vi "Main.vi"() -> ()   [LabVIEW 2023]
doc: "This template is for the Queued Message Handler design pattern.\n\nThe Event Handling Loop generates messages based on user interface actions.\n\nThe Message Handling Loop processes messages generated by the Event Handling Loop, or by other messages. The messages are string values, so new messages can be added easily to the Message Cases case structure in the Message Handling Loop. Each message cluster can also provide an optional value for Message Data, which is a variant that can be converted to whatever message-specific data is required."
uses:
  controls/UI Data.ctl
  support/Message Queue/Enqueue Message (Single).vi
  <vilib>/Utility/file.llb/Write Delimited Spreadsheet (string).vi
  <vilib>/Utility/file.llb/Write Delimited Spreadsheet (DBL).vi
  <vilib>/Instr/_visa.llb/VISA Configure Serial Port (Instr).vi
  <vilib>/Utility/error.llb/Error Cluster From Error Code.vi
  <vilib>/ErrorRing/Error Ring.xnode
  support/Message Queue/Message Queue.lvlib
  support/User Event - Stop/User Event - Stop.lvlib
panel:
  in  "File Path":path
  in  "Test Name":string
  out "Torque vs Displacement":cluster{dbl[], dbl[]}(graph)
  in  "VISA resource name":refnum<visa-resource-name>
  in  "Cycles":dbl
  in  "Torque":dbl
  in  "Microsteps":dbl
  in  "RPM":dbl
  in  "Clear":bool
  in  "Save":bool
  out "Status":string
  in  "Stop":bool
  in  "Start":bool
  in  "Exit":bool
  # "Torque vs Displacement"
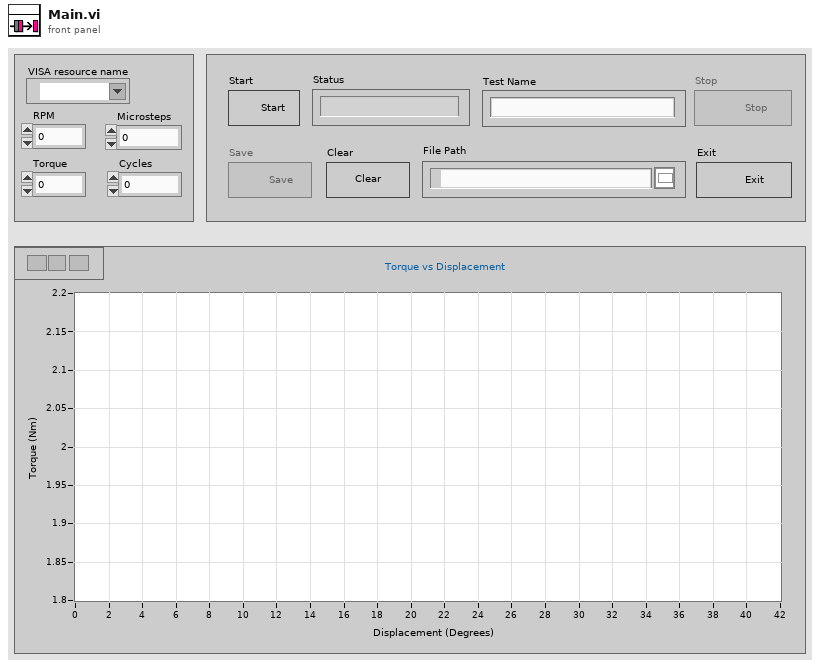
[diagram p1: front panel]
types:
  T1 = cluster{"RPM":dbl, "Microsteps":dbl, "Torque":dbl, "Cycles":dbl, "VISA resource name":refnum<visa-resource-name>}
  T2 = typedef "UI Data.ctl" = cluster{"Start ref":refnum<vi>, "Stop ref":refnum<vi>, "Status ref":refnum<vi>, "Exit ref":refnum<vi>, "Save ref":refnum<vi>, "Clear ref":refnum<vi>}
  T3 = typedef "Message Queue.lvlib/All Message Queues.ctl" = cluster{"UI":refnum<queue>, "Acquisition":refnum<queue>}
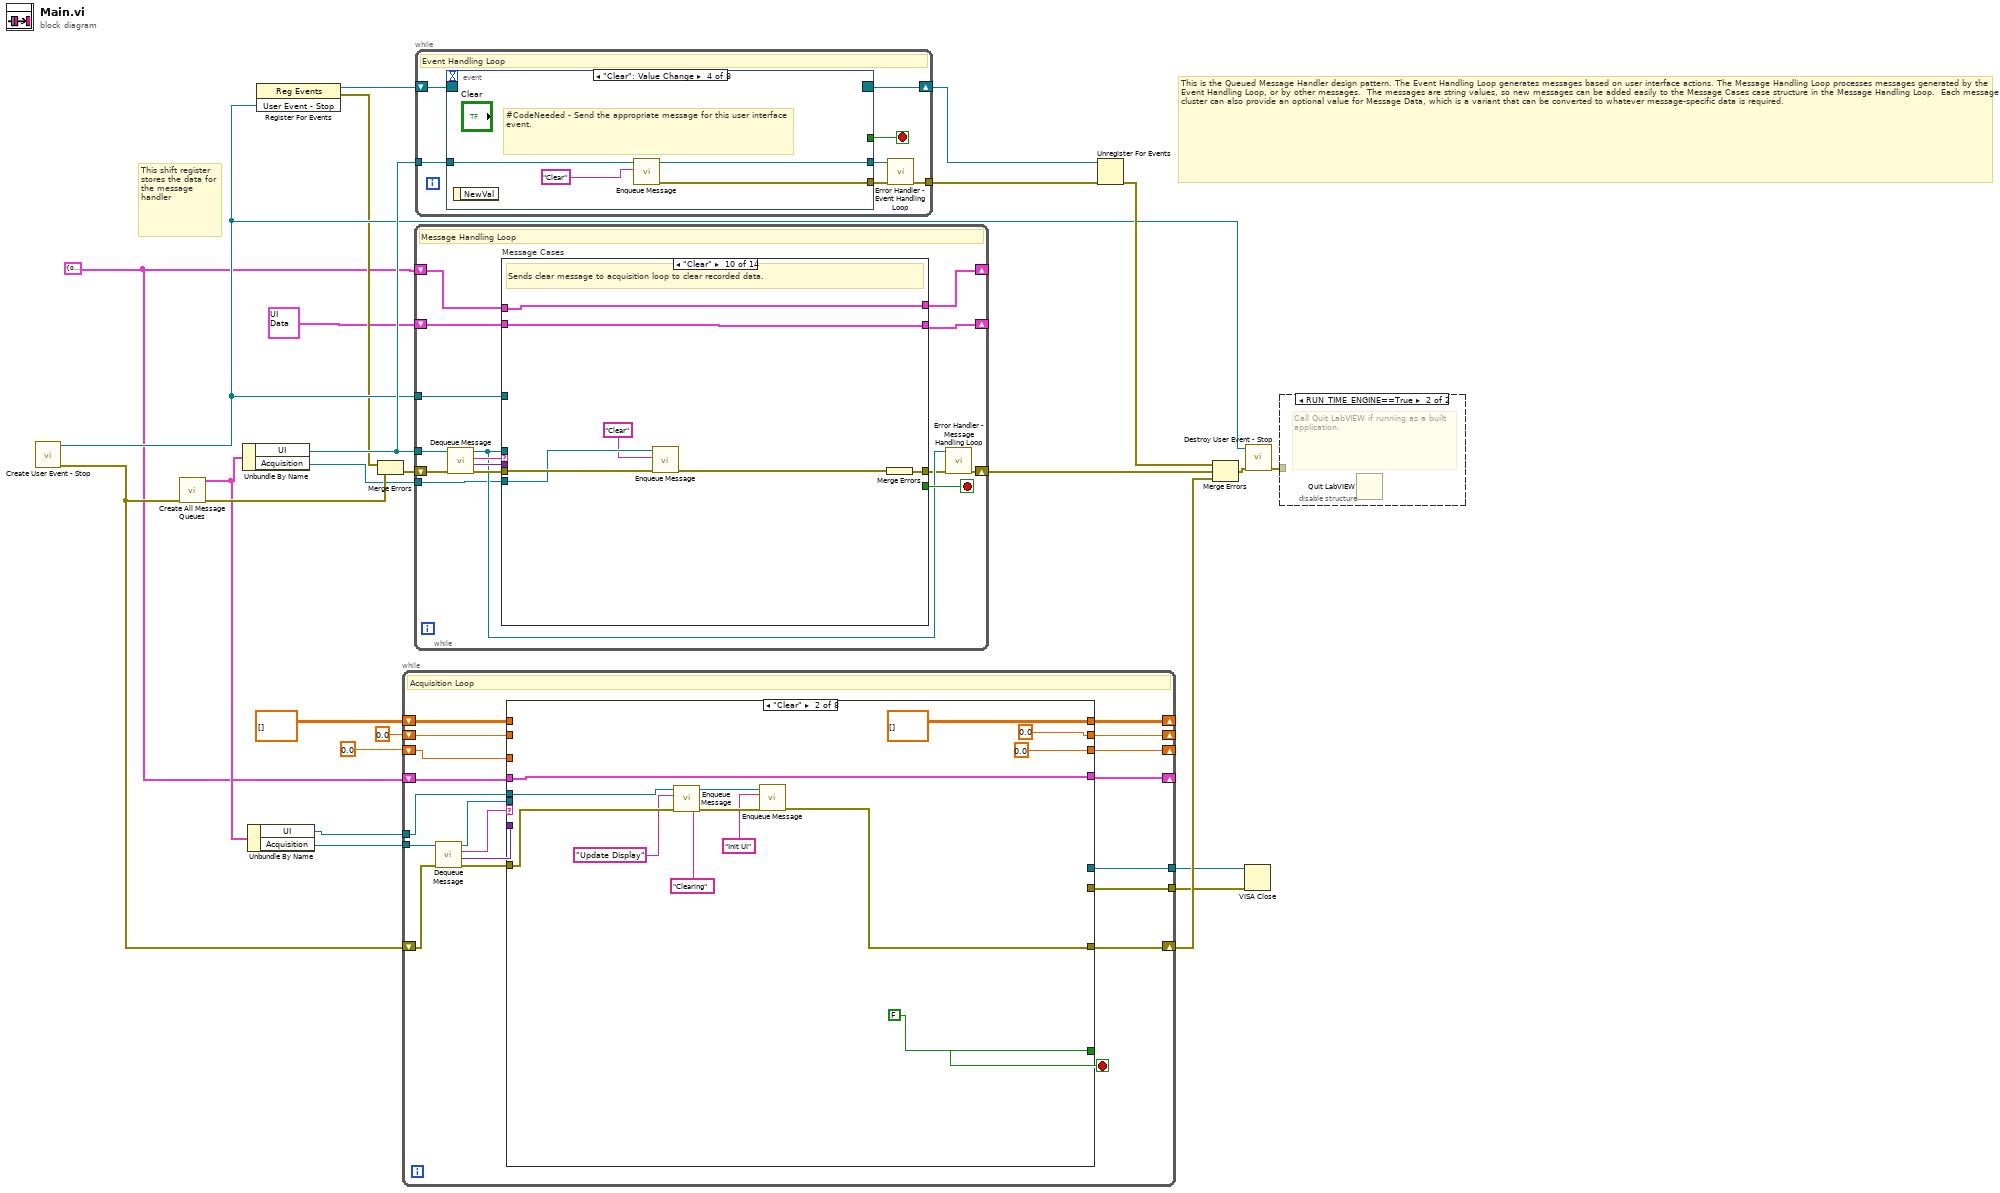
[diagram p0: block diagram]
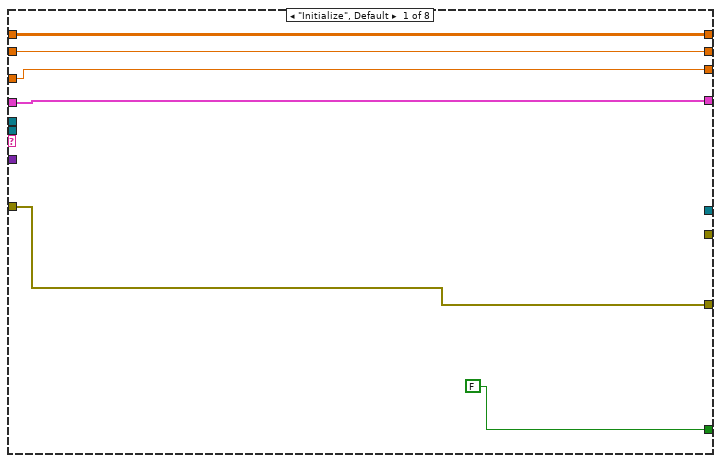
[diagram p2: hidden frame]
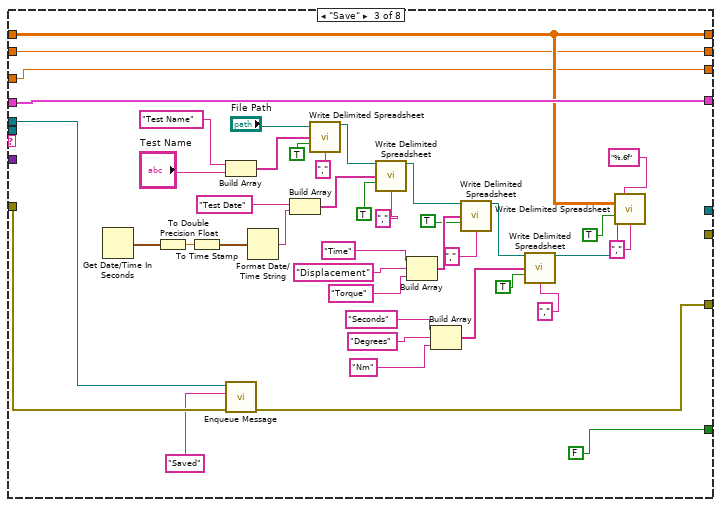
[diagram p3: hidden frame]
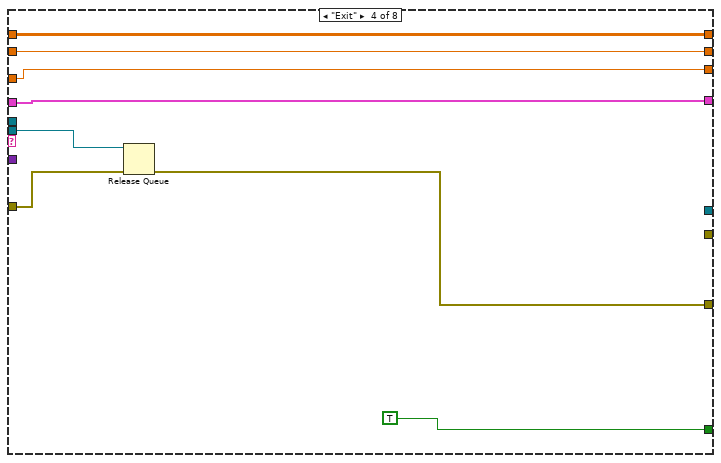
[diagram p4: hidden frame]
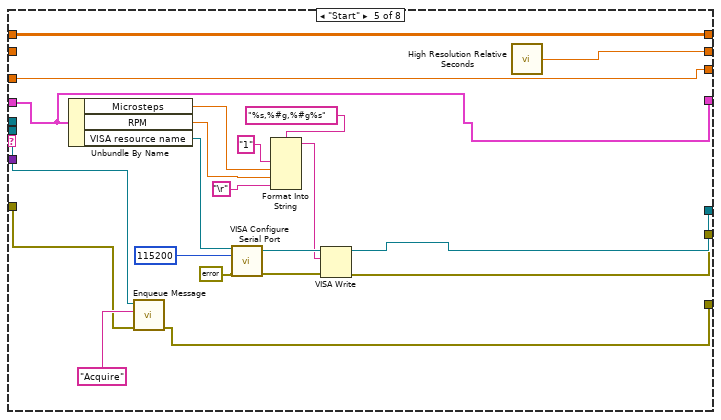
[diagram p5: hidden frame]
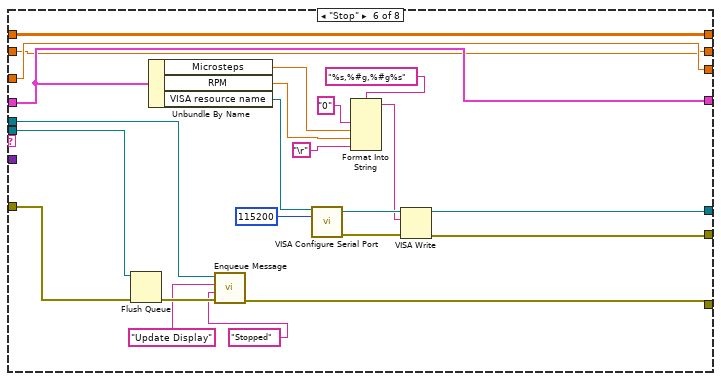
[diagram p6: hidden frame]
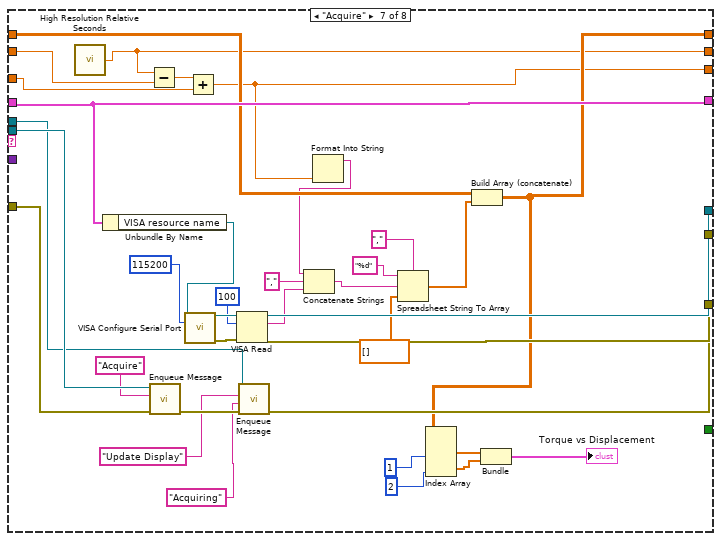
[diagram p7: hidden frame]
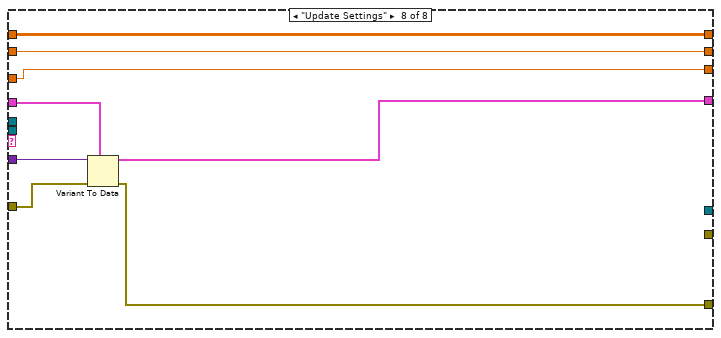
[diagram p8: hidden frame]
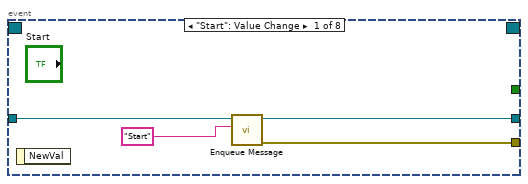
[diagram p10: hidden frame]
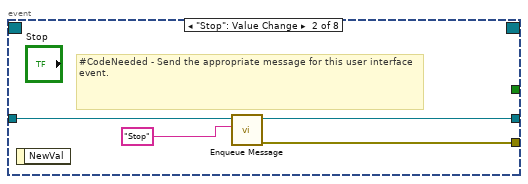
[diagram p11: hidden frame]
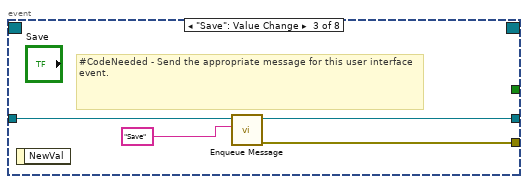
[diagram p12: hidden frame]
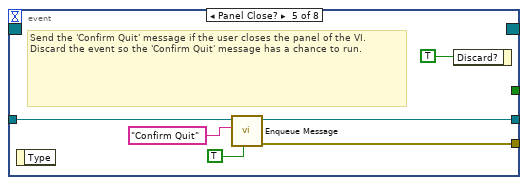
[diagram p13: hidden frame]
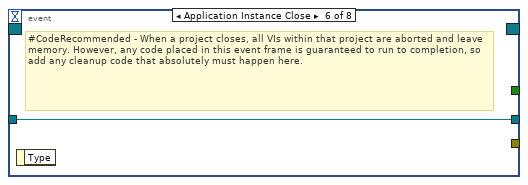
[diagram p14: hidden frame]
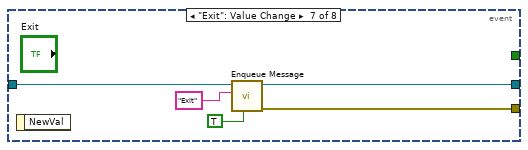
[diagram p15: hidden frame]
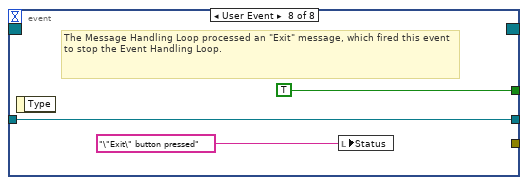
[diagram p16: hidden frame]
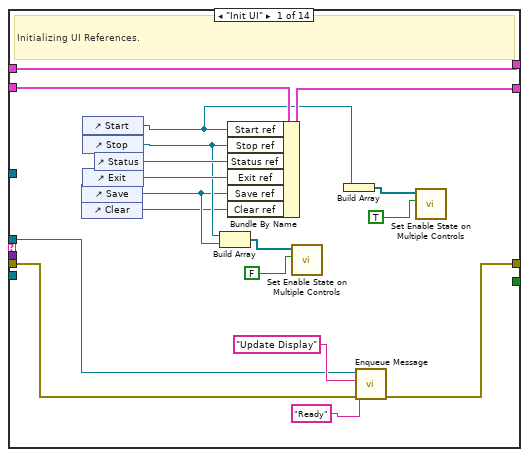
[diagram p17: hidden frame]
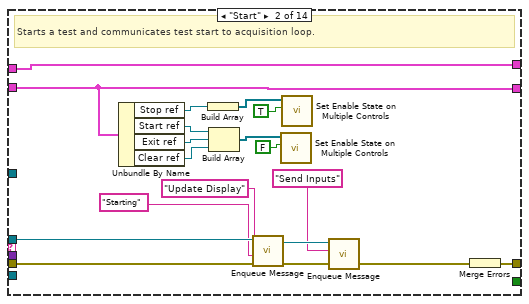
[diagram p18: hidden frame]
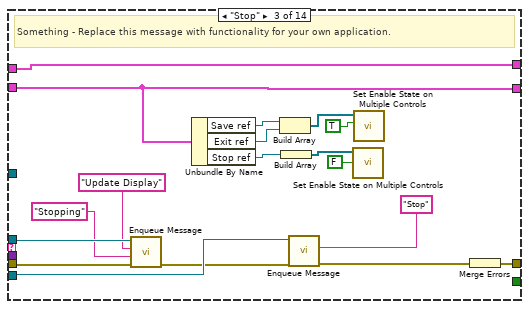
[diagram p19: hidden frame]
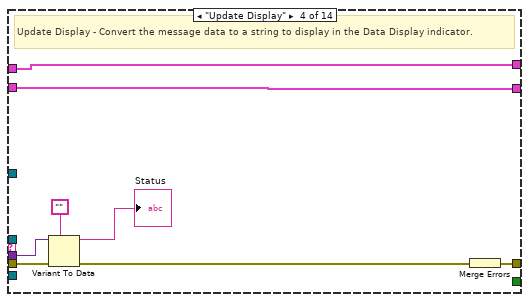
[diagram p20: hidden frame]
diagram:
  w8 = T1 {"RPM"=0.0, "Microsteps"=0.0, "Torque"=0.0, "Cycles"=0.0, "VISA resource name"=""}
  # "This is the Queued Message Handler design pattern. The Event Handling Loop generates messages based on user interface actions. The Message Handling Loop processes messages generated by the Event Handling Loop, or by other messages.  The messages are string values, so new messages can be added easily to the Message Cases case structure in the Message Handling Loop.  Each message cluster can also provide an optional value for Message Data, which is a variant that can be converted to whatever message-specific data is required."
  # "This shift register stores the data for the message handler"
  n1 = call "Create User Event - Stop.vi"() -> ("error out"=w9:errorcluster, "User Event - Stop"=w16:refnum<user-event>)  [unwired: 10 in]
  n2 = call "Create All Message Queues.vi"("error in (no error)"=w9) -> ("error out"=w25:errorcluster, "Message Queues out"=w11:T3)  [unwired: 9 in]
  n3 = Unbundle By Name(w11) -> ("UI"=w23:refnum<queue>, "Acquisition"=w12:refnum<queue>)
  n4 = Unbundle By Name(w11) -> ("UI"=w7:refnum<queue>, "Acquisition"=w10:refnum<queue>)
  n5 = register-events(w16) -> (reference out=w17:refnum<event-registration>, error out=w14:errorcluster)  [unwired: 2 in]
  n6 = Merge Errors(w14, w25) -> (w15:errorcluster)
  n7 = while {
    tunnel: w10 -> [w44]
    shift-right: [w32] -> w6
    shift-left: w9 -> [w43]
    shift-right: [w38] -> _
    shift-left: w8 -> [w41]
    tunnel: w7 -> [w33]
    tunnel: [w35] -> w5
    tunnel: [w34] -> w4
    shift-right: [w30] -> _
    shift-left: dbl[][] [] -> [w31]
    shift-right: [w29] -> _
    shift-left: 0.0 -> [w28]
    shift-right: [w27] -> _
    shift-left: 0.0 -> [w26]
    stop <- w37 stop-if-true
    # "Acquisition Loop"
    n8 = call "Dequeue Message.vi"("error in (no error)"=w43, "Message Queue"=w44) -> ("error out"=w42:errorcluster, "Message Data"=w39:variant, "Message"=w40:string, "dup Message Queue"=w36:refnum<queue>)  [unwired: 6 in]
    n9 = case shown="\"Clear\"" w40 {
      tunnel: w42 -> [w48 w61 w102 w110 w121 w142 w185 w199]
      tunnel: w41 -> [w50 w63 w105 w113 w124 w147 w191 w200]
      tunnel: w39 -> [_ _ _ _ _ _ _ w201]
      tunnel: [w50 w63 w105 w113 w124 w147 w191 w198] -> w38
      tunnel: [FALSE FALSE FALSE TRUE _ _ _ _] -> w37
      tunnel: w36 -> [_ _ _ w111 w118 w143 w186 _]
      tunnel: [_ _ _ _ w122 w146 w188 _] -> w35
      tunnel: [_ _ _ _ w120 w145 w187 _] -> w34
      tunnel: w33 -> [_ w60 w103 _ _ w139 w181 _]
      tunnel: [w48 w55 w64 w109 w117 w140 w182 w197] -> w32
      tunnel: w31 -> [w47 _ w97 w108 w116 w144 w174 w196]
      tunnel: [w47 dbl[][] [] w97 w108 w116 w144 w163 w196] -> w30
      tunnel: [w46 0.0 w78 w107 w115 w137 w159 w195] -> w29
      tunnel: w28 -> [w46 _ w78 w107 w115 w137 w162 w195]
      tunnel: [w45 0.0 w75 w106 w114 w136 w158 w194] -> w27
      tunnel: w26 -> [w45 _ w75 w106 _ w136 w161 w194]
      frame "Initialize", Default {
      }
      frame "Clear" {
        n10 = call-poly "Enqueue Message.vi"("error in (no error)"=w61, "Message Data"="Clearing" ("Message"), "Message"="Update Display", "Message Queue"=w60) -> ("error out"=w56:errorcluster, "dup Message Queue"=w57:refnum<queue>)  [unwired: 6 in]
        n11 = call-poly "Enqueue Message.vi"("error in (no error)"=w56, "Message"="Init UI", "Message Queue"=w57) -> ("error out"=w55:errorcluster)  [unwired: 7 in, 1 out]
      }
      frame "Save" {
        n12 = Get Date/Time In Seconds() -> (seconds since 1Jan1904=w73:timestamp)
        n13 = To Double Precision Float(number=w73) -> (double precision float=w74:dbl)
        n14 = To Time Stamp(1:w74) -> (0:w70:timestamp)
        n15 = Build Array("Test Name" ("delimiter (\\t)"), "Test Name") -> (w95:string[])
        n16 = call-poly "Enqueue Message.vi"("error in (no error)"=w102, "Message"="Saved", "Message Queue"=w103) -> ("error out"=w64:errorcluster)  [unwired: 7 in, 1 out]
        n17 = Format Date/Time String(seconds (now)=w70) -> (date/time string=w66:string)  [unwired: 2 in]
        n18 = Build Array("Test Date" ("delimiter (\\t)"), w66) -> (w65:string[])
        n19 = call-poly <vilib>:"Write Delimited Spreadsheet.vi"("file path (dialog if empty)"="File Path", "1D data"=w95, "append to file? (new file:F)"=TRUE, "delimiter (\\t)"="," ("delimiter (\\t)")) -> ("new file path (Not A Path if cancelled)"=w69:path)  [unwired: 10 in, 1 out]
        n20 = call-poly <vilib>:"Write Delimited Spreadsheet.vi"("file path (dialog if empty)"=w69, "1D data"=w65, "append to file? (new file:F)"=TRUE, "delimiter (\\t)"="," ("delimiter (\\t)")) -> ("new file path (Not A Path if cancelled)"=w68:path)  [unwired: 10 in, 1 out]
        n21 = Build Array("Time" ("element"), "Displacement" ("delimiter (\\t)"), "Torque" ("delimiter (\\t)")) -> (w89:string[])
        n22 = Build Array("Seconds" ("element"), "Degrees" ("delimiter (\\t)"), "Nm" ("delimiter (\\t)")) -> (w88:string[])
        n23 = call-poly <vilib>:"Write Delimited Spreadsheet.vi"("file path (dialog if empty)"=w68, "1D data"=w89, "append to file? (new file:F)"=TRUE, "delimiter (\\t)"="," ("delimiter (\\t)")) -> ("new file path (Not A Path if cancelled)"=w87:path)  [unwired: 10 in, 1 out]
        n24 = call-poly <vilib>:"Write Delimited Spreadsheet.vi"("file path (dialog if empty)"=w87, "1D data"=w88, "append to file? (new file:F)"=TRUE, "delimiter (\\t)"="," ("delimiter (\\t)")) -> ("new file path (Not A Path if cancelled)"=w86:path)  [unwired: 10 in, 1 out]
        n25 = call-poly <vilib>:"Write Delimited Spreadsheet.vi"("file path (dialog if empty)"=w86, "format (%.3f)"="%.6f", "2D data"=w97, "append to file? (new file:F)"=TRUE, "delimiter (\\t)"="," ("delimiter (\\t)")) -> ()  [unwired: 9 in, 2 out]
      }
      frame "Exit" {
        n26 = Release Queue(queue=w111, error in (no error)=w110) -> (error out=w109:errorcluster)  [unwired: 1 in, 2 out]
      }
      frame "Start" {
        n27 = Unbundle By Name(w124) -> ("Microsteps"=w131:dbl, "RPM"=w130:dbl, "VISA resource name"=w129:refnum<visa-resource-name>)
        n28 = call-poly "Enqueue Message.vi"("error in (no error)"=w121, "Message"="Acquire", "Message Queue"=w118) -> ("error out"=w117:errorcluster)  [unwired: 7 in, 1 out]
        n29 = call-poly "VISA Configure Serial Port"("VISA resource name"=w129, "baud rate (9600)"=u32 115200, "error in (no error)"=errorcluster {"status"=FALSE, "code"=0, "source"=""}) -> ("VISA resource name out"=w126:refnum<visa-resource-name>, "error out"=w127:errorcluster)  [unwired: 11 in]
        n30 = Format Into String(format string="%s,%#g,%#g%s", "1", w131, w130, "\r") -> (resulting string=w125:string)  [unwired: 2 in, 1 out]
        n31 = VISA Write(VISA resource name=w126, write buffer=w125, error in (no error)=w127) -> (VISA resource name out=w122:refnum<visa-resource-name>, error out=w120:errorcluster)  [unwired: 1 out]
        n32 = call <vilib>:"High Resolution Relative Seconds.vi"() -> ("relative seconds"=w114:dbl)
      }
      frame "Stop" {
        n33 = Flush Queue(queue=w143, error in (no error)=w142) -> (error out=w141:errorcluster)  [unwired: 2 out]
        n34 = Unbundle By Name(w147) -> ("Microsteps"=w154:dbl, "RPM"=w153:dbl, "VISA resource name"=w152:refnum<visa-resource-name>)
        n35 = call-poly "Enqueue Message.vi"("error in (no error)"=w141, "Message Data"="Stopped" ("Message"), "Message"="Update Display", "Message Queue"=w139) -> ("error out"=w140:errorcluster)  [unwired: 6 in, 1 out]
        n36 = call-poly "VISA Configure Serial Port"("VISA resource name"=w152, "baud rate (9600)"=u32 115200) -> ("VISA resource name out"=w149:refnum<visa-resource-name>, "error out"=w150:errorcluster)  [unwired: 12 in]
        n37 = Format Into String(format string="%s,%#g,%#g%s", "0", w154, w153, "\r") -> (resulting string=w148:string)  [unwired: 2 in, 1 out]
        n38 = VISA Write(VISA resource name=w149, write buffer=w148, error in (no error)=w150) -> (VISA resource name out=w146:refnum<visa-resource-name>, error out=w145:errorcluster)  [unwired: 1 out]
      }
      frame "Acquire" {
        n39 = call <vilib>:"High Resolution Relative Seconds.vi"() -> ("relative seconds"=w158:dbl)
        n40 = Unbundle By Name(w191) -> ("VISA resource name"=w193:refnum<visa-resource-name>)
        n41 = Subtract(x=w158, y=w161) -> (x-y=w160:dbl)
        n42 = call-poly "Enqueue Message.vi"("error in (no error)"=w185, "Message"="Acquire", "Message Queue"=w186) -> ("error out"=w183:errorcluster)  [unwired: 7 in, 1 out]
        n43 = call-poly "VISA Configure Serial Port"("VISA resource name"=w193, "baud rate (9600)"=u32 115200) -> ("VISA resource name out"=w190:refnum<visa-resource-name>, "error out"=w189:errorcluster)  [unwired: 12 in]
        n44 = Add(x=w160, y=w162) -> (x+y=w159:dbl)
        n45 = VISA Read(VISA resource name=w190, byte count=u32 100, error in (no error)=w189) -> (VISA resource name out=w188:refnum<visa-resource-name>, read buffer=w165:string, error out=w187:errorcluster)  [unwired: 1 out]
        n46 = call-poly "Enqueue Message.vi"("error in (no error)"=w183, "Message Data"="Acquiring" ("\"Do Something\" button pressed"), "Message"="Update Display", "Message Queue"=w181) -> ("error out"=w182:errorcluster)  [unwired: 6 in, 1 out]
        n47 = Format Into String(w159) -> (resulting string=w164:string)  [unwired: 3 in, 1 out]
        n48 = Concatenate Strings(w164, "," ("string"), w165) -> (w166:string)
        n49 = Spreadsheet String To Array(delimiter (Tab)=",", format string="%d", spreadsheet string=w166, array type (2D Dbl)=dbl[] []) -> (array=w173:dbl[])
        n50 = Build Array (concatenate)(w174, w173) -> (w163:dbl[][])
        n51 = Index Array(array=w163, index (col) #1=1 ("index (col)"), index (col) #2=2 ("index (col)")) -> (element #1=w170:dbl[], element #2=w169:dbl[])  [unwired: 2 in]
        n52 = Bundle(w170, w169) -> (→"Torque vs Displacement":cluster{dbl[], dbl[]})  [unwired: 1 in]
      }
      frame "Update Settings" {
        n53 = Variant To Data(error in=w199, type=w200, Variant=w201) -> (data=w198:T1, error out=w197:errorcluster)
      }
    }
  }
  n54 = while {
    tunnel: w23 -> [w208]
    shift-right: [w215] -> _
    shift-left: T2 {"Start ref"=refnum, "Stop ref"=refnum, "Status ref"=refnum, "Exit ref"=refnum, "Save ref"=refnum, "Clear ref"=refnum} ("Data Cluster") -> [w216]
    tunnel: w16 -> [w213]
    shift-right: [w204] -> _
    shift-left: w8 -> [w203]
    tunnel: w12 -> [w202]
    shift-right: [w206] -> w24
    shift-left: w15 -> [w212]
    stop <- w214 stop-if-true
    # "Message Handling Loop"
    n55 = call "Dequeue Message.vi"("error in (no error)"=w212, "Message Queue"=w208) -> ("error out"=w211:errorcluster, "Message Data"=w209:variant, "Message"=w210:string, "dup Message Queue"=w207:refnum<queue>)  [unwired: 6 in]
    n56 = case "Message Cases" shown="\"Clear\"" w210 {
      selector: w210 -> [_ _ _ _ _ _ _ _ _ _ _ _ _ w364]
      tunnel: w207 -> [w226 w251 w264 _ _ w291 _ w303 w315 _ _ _ w362 _]
      tunnel: w211 -> [w225 w252 w266 w277 w287 w295 w299 w304 w316 w323 w330 w342 w355 _]
      tunnel: [w234 w253 w271 w278 w281 w293 w297 w313 w319 w326 w333 w349 w358 w365] -> w205
      tunnel: w216 -> [w233 w241 w255 w279 w286 w294 w298 w305 w320 w327 w334 w350 w361 w366]
      tunnel: [w232 w241 w255 w279 w286 w294 w298 w305 w320 w327 w334 w350 w361 w366] -> w215
      tunnel: [_ _ _ _ _ _ _ _ _ _ _ _ TRUE _] -> w214
      tunnel: w209 -> [_ _ _ w276 w285 _ _ _ _ _ _ _ _ _]
      tunnel: w213 -> [_ _ _ _ _ _ _ _ _ _ _ _ w357 _]
      tunnel: w203 -> [w227 w248 w270 w272 w280 w288 w296 w312 w318 w325 w332 w348 w351 w363]
      tunnel: [w227 w248 w270 w272 w280 w288 w296 w312 w318 w325 w332 w341 w351 w363] -> w204
      tunnel: w202 -> [_ _ w267 _ _ _ _ _ _ w322 w329 w339 w354 _]
      frame "Init UI" {
        # "Initializing UI References."
        n57 = control-ref of="Save"() -> (w221:refnum<vi>)
        n58 = control-ref of="Clear"() -> (w220:refnum<vi>)
        n59 = control-ref of="Start"() -> (w217:refnum<vi>)
        n60 = control-ref of="Stop"() -> (w222:refnum<vi>)
        n61 = control-ref of="Exit"() -> (w230:refnum<vi>)
        n62 = control-ref of="Status"() -> (w231:refnum<vi>)
        n63 = Build Array(w222, w221) -> (w223:refnum<vi>[])
        n64 = Bundle By Name(cluster=w233, "Start ref"=w217, "Stop ref"=w222, "Status ref"=w231, "Exit ref"=w230, "Save ref"=w221, "Clear ref"=w220) -> (w232:T2)
        n65 = call "Set Enable State on Multiple Controls.vi"("Enable?"=FALSE, "Controls"=w223) -> ()  [unwired: 10 in]
        n66 = Build Array(w217) -> (w218:refnum<vi>[])
        n67 = call-poly "Enqueue Message.vi"("error in (no error)"=w225, "Message Data"="Ready" ("Initial Message"), "Message"="Update Display", "Message Queue"=w226) -> ("error out"=w234:errorcluster)  [unwired: 6 in, 1 out]
        n68 = call "Set Enable State on Multiple Controls.vi"("Enable?"=TRUE, "Controls"=w218) -> ()  [unwired: 10 in]
      }
      frame "Start" {
        # "Starts a test and communicates test start to acquisition loop."
        n69 = Unbundle By Name(w241) -> ("Stop ref"=w238:refnum<vi>, "Start ref"=w236:refnum<vi>, "Exit ref"=w240:refnum<vi>, "Clear ref"=w235:refnum<vi>)
        n70 = Build Array(w238) -> (w237:refnum<vi>[])
        n71 = Build Array(w236, w240, w235) -> (w242:refnum<vi>[])
        n72 = call-poly "Enqueue Message.vi"("error in (no error)"=w252, "Message Data"="Starting" ("\"Do Something\" button pressed"), "Message"="Update Display", "Message Queue"=w251) -> ("error out"=w247:errorcluster, "dup Message Queue"=w246:refnum<queue>)  [unwired: 6 in]
        n73 = call "Set Enable State on Multiple Controls.vi"("Enable?"=FALSE, "Controls"=w242) -> ()  [unwired: 10 in]
        n74 = call "Set Enable State on Multiple Controls.vi"("Enable?"=TRUE, "Controls"=w237) -> ()  [unwired: 10 in]
        n75 = call-poly "Enqueue Message.vi"("error in (no error)"=w247, "Message"="Send Inputs", "Message Queue"=w246) -> ("error out"=w244:errorcluster)  [unwired: 7 in, 1 out]
        n76 = Merge Errors(w244) -> (w253:errorcluster)
      }
      frame "Stop" {
        # "Something - Replace this message with functionality for your own application."
        n77 = call-poly "Enqueue Message.vi"("error in (no error)"=w266, "Message Data"="Stopping" ("Message"), "Message"="Update Display", "Message Queue"=w264) -> ("error out"=w265:errorcluster)  [unwired: 6 in, 1 out]
        n78 = Unbundle By Name(w255) -> ("Save ref"=w260:refnum<vi>, "Exit ref"=w254:refnum<vi>, "Stop ref"=w259:refnum<vi>)
        n79 = Build Array(w260, w254) -> (w261:refnum<vi>[])
        n80 = Build Array(w259) -> (w258:refnum<vi>[])
        n81 = call-poly "Enqueue Message.vi"("error in (no error)"=w265, "Message"="Stop", "Message Queue"=w267) -> ("error out"=w269:errorcluster)  [unwired: 7 in, 1 out]
        n82 = call "Set Enable State on Multiple Controls.vi"("Enable?"=FALSE, "Controls"=w258) -> ()  [unwired: 10 in]
        n83 = call "Set Enable State on Multiple Controls.vi"("Enable?"=TRUE, "Controls"=w261) -> ()  [unwired: 10 in]
        n84 = Merge Errors(w269) -> (w271:errorcluster)
      }
      frame "Update Display" {
        # "Update Display - Convert the message data to a string to display in the Data Display indicator."
        n85 = Variant To Data(error in=w277, type="", Variant=w276) -> (data=→"Status":string, error out=w274:errorcluster)
        n86 = Merge Errors(w274) -> (w278:errorcluster)
      }
      frame "Error" {
        # "Error - Display an error dialog. This message is sent by the \"Error Handler\" VIs at the end of other loops in this application."
        n87 = Variant To Data(error in=w287, type=errorcluster {"status"=FALSE, "code"=0, "source"=""} ("error constant"), Variant=w285) -> (data=w283:errorcluster, error out=w282:errorcluster)
        n88 = call <vilib>:"Simple Error Handler.vi"("error in (no error)"=w283) -> ()  [unwired: 4 in, 5 out]
        n89 = Merge Errors(w282) -> (w281:errorcluster)
      }
      frame "Confirm Quit" {
        # "#CodeNeeded - If you want to provide an \"Are you sure\" dialog (or some other notification) before the application exits, place that code here. This message is typically sent from a Panel Close? event."
        # "Confirm Quit - Message that can confirm whether or not the user wants to exit the application."
        n90 = call-poly "Enqueue Message.vi"("Priority Message? (F)"=TRUE, "error in (no error)"=w295, "Message"="Exit", "Message Queue"=w291) -> ("error out"=w292:errorcluster)  [unwired: 6 in, 1 out]
        n91 = Merge Errors(w292) -> (w293:errorcluster)
      }
      frame "---Copy This Frame---" {
        # "Duplicate this frame when creating new messages.  Change this comment in the duplicated frame to describe this message."
        n92 = Merge Errors(w299) -> (w297:errorcluster)
      }
      frame "Saved" {
        # "Duplicate this frame when creating new messages.  Change this comment in the duplicated frame to describe this message."
        n93 = call-poly "Enqueue Message.vi"("error in (no error)"=w304, "Message Data"="Saved" ("Message"), "Message"="Update Display", "Message Queue"=w303) -> ("error out"=w300:errorcluster)  [unwired: 6 in, 1 out]
        n94 = Unbundle By Name(w305) -> ("Clear ref"=w311:refnum<vi>, "Save ref"=w309:refnum<vi>)
        n95 = Build Array(w311) -> (w308:refnum<vi>[])
        n96 = Build Array(w309) -> (w310:refnum<vi>[])
        n97 = call "Set Enable State on Multiple Controls.vi"("Enable?"=TRUE, "Controls"=w308) -> ()  [unwired: 10 in]
        n98 = call "Set Enable State on Multiple Controls.vi"("Enable?"=FALSE, "Controls"=w310) -> ()  [unwired: 10 in]
        n99 = Merge Errors(w300) -> (w313:errorcluster)
      }
      frame "Initialize" {
        # "Duplicate this frame when creating new messages.  Change this comment in the duplicated frame to describe this message."
        n100 = call-poly "Enqueue Message.vi"("error in (no error)"=w316, "Message"="Init UI", "Message Queue"=w315) -> ("error out"=w317:errorcluster)  [unwired: 7 in, 1 out]
        n101 = Merge Errors(w317) -> (w319:errorcluster)
      }
      frame "Clear" {
        # "Sends clear message to acquisition loop to clear recorded data."
        n102 = call-poly "Enqueue Message.vi"("error in (no error)"=w323, "Message"="Clear", "Message Queue"=w322) -> ("error out"=w324:errorcluster)  [unwired: 7 in, 1 out]
        n103 = Merge Errors(w324) -> (w326:errorcluster)
      }
      frame "Save" {
        # "Saves Current Data"
        n104 = call-poly "Enqueue Message.vi"("error in (no error)"=w330, "Message"="Save", "Message Queue"=w329) -> ("error out"=w331:errorcluster)  [unwired: 7 in, 1 out]
        n105 = Merge Errors(w331) -> (w333:errorcluster)
      }
      frame "Send Inputs" {
        # "Send updated inputs to acquistion loop."
        n106 = Bundle By Name(cluster=w348, "RPM"="RPM", "Microsteps"="Microsteps", "Torque"="Torque", "Cycles"="Cycles", "VISA resource name"="VISA resource name") -> (w341:T1)
        n107 = call-poly "Enqueue Message.vi"("error in (no error)"=w342, "Message Data"=w341, "Message"="Update Settings", "Message Queue"=w339) -> ("error out"=w337:errorcluster, "dup Message Queue"=w335:refnum<queue>)  [unwired: 6 in]
        n108 = call-poly "Enqueue Message.vi"("error in (no error)"=w337, "Message"="Start", "Message Queue"=w335) -> ("error out"=w336:errorcluster)  [unwired: 7 in, 1 out]
        n109 = Merge Errors(w336) -> (w349:errorcluster)
      }
      frame "Exit" {
        # "Stop the VI"
        # "Release the message queue reference"
        # "Exit - Exit the application."
        n110 = call-poly "Enqueue Message.vi"("Priority Message? (F)"=TRUE, "Message"="Exit", "Message Queue"=w354) -> ()  [unwired: 7 in, 2 out]
        n111 = call "Fire User Event - Stop.vi"("User Event - Stop"=w357) -> ("error out"=w356:errorcluster)  [unwired: 10 in]
        n112 = Release Queue(queue=w362, error in (no error)=w355) -> (error out=w359:errorcluster)  [unwired: 1 in, 2 out]
        n113 = Merge Errors(w356, w359) -> (w358:errorcluster)
      }
      frame Default {
        # "'Default' case only runs if there is a message that isn't defined in any of the other cases.  Output a programming error."
        n114 = xnode "Error Ring"("parameter 0"=w364) -> ("error out"=w365:errorcluster)
      }
    }
    n115 = call "Error Handler - Message Handling Loop.vi"("error in (no error)"=w205, "Message Queue"=w207) -> ("dup error in"=w206:errorcluster)  [unwired: 8 in, 1 out]
  }
  n116 = while {
    tunnel: w23 -> [w380]
    shift-right: [w378] -> w20
    shift-left: w17 -> [w379]
    tunnel: [w374] -> w18
    stop <- w376 stop-if-true
    # "Event Handling Loop"
    n117 = event shown="[3] \"Clear\": Value Change" {
      selector: w379 -> [_ _ _ _ _ _ _ _]
      dyn-events: [_ _ _ _ _ _ _ _] -> w378
      timeout: _ -> [_ _ _ _ _ _ _ _]
      tunnel: [_ _ _ _ _ _ _ TRUE ("Discard?")] -> w376
      tunnel: w380 -> [w384 w388 w392 w396 w401 w403 w408 w411]
      tunnel: [w381 w385 w389 w393 w400 _ w407 _] -> w377
      tunnel: [w383 w387 w391 w395 w399 w403 w406 w411] -> w375
      event "Start": Value Change {
        n118 = event-data() -> ()  [unwired: 1 in, 1 out]
        n119 = call-poly "Enqueue Message.vi"("Message"="Start", "Message Queue"=w384) -> ("error out"=w381:errorcluster, "dup Message Queue"=w383:refnum<queue>)  [unwired: 8 in]
      }
      event "Stop": Value Change {
        # "#CodeNeeded - Send the appropriate message for this user interface event."
        n120 = event-data() -> ()  [unwired: 1 in, 1 out]
        n121 = call-poly "Enqueue Message.vi"("Message"="Stop", "Message Queue"=w388) -> ("error out"=w385:errorcluster, "dup Message Queue"=w387:refnum<queue>)  [unwired: 8 in]
      }
      event "Save": Value Change {
        # "#CodeNeeded - Send the appropriate message for this user interface event."
        n122 = event-data() -> ()  [unwired: 1 in, 1 out]
        n123 = call-poly "Enqueue Message.vi"("Message"="Save", "Message Queue"=w392) -> ("error out"=w389:errorcluster, "dup Message Queue"=w391:refnum<queue>)  [unwired: 8 in]
      }
      event "Clear": Value Change {
        # "#CodeNeeded - Send the appropriate message for this user interface event."
        n124 = event-data() -> ()  [unwired: 1 in, 1 out]
        n125 = call-poly "Enqueue Message.vi"("Message"="Clear", "Message Queue"=w396) -> ("error out"=w393:errorcluster, "dup Message Queue"=w395:refnum<queue>)  [unwired: 8 in]
      }
      event Panel Close? {
        # "Send the 'Confirm Quit' message if the user closes the panel of the VI. Discard the event so the 'Confirm Quit' message has a chance to run."
        n126 = event-data() -> ()  [unwired: 1 in, 1 out]
        n127 = call-poly "Enqueue Message.vi"("Priority Message? (F)"=TRUE, "Message"="Confirm Quit", "Message Queue"=w401) -> ("error out"=w400:errorcluster, "dup Message Queue"=w399:refnum<queue>)  [unwired: 7 in]
        n128 = event-data("Discard?"=TRUE) -> ()  [unwired: 1 in, 1 out]
      }
      event Application Instance Close {
        # "#CodeRecommended - When a project closes, all VIs within that project are aborted and leave memory. However, any code placed in this event frame is guaranteed to run to completion, so add any cleanup code that absolutely must happen here."
        n129 = event-data() -> ()  [unwired: 1 in, 1 out]
      }
      event "Exit": Value Change {
        n130 = event-data() -> ()  [unwired: 1 in, 1 out]
        n131 = call-poly "Enqueue Message.vi"("Priority Message? (F)"=TRUE, "Message"="Exit", "Message Queue"=w408) -> ("error out"=w407:errorcluster, "dup Message Queue"=w406:refnum<queue>)  [unwired: 7 in]
      }
      event User Event {
        # "The Message Handling Loop processed an \"Exit\" message, which fired this event to stop the Event Handling Loop."
        n132 = event-data() -> ()  [unwired: 1 in, 1 out]
        n133 = local write "Status"("\"Exit\" button pressed" ("VI Stopped")) -> ()
      }
    }
    n134 = call "Error Handler - Event Handling Loop.vi"("error in (no error)"=w377, "Message Queue"=w375) -> ("dup error in"=w374:errorcluster)  [unwired: 8 in, 1 out]
  }
  n135 = Unregister For Events(event registration refnum=w20, error in=w18) -> (error out=w21:errorcluster)
  n136 = Merge Errors(w21, w24, w6) -> (w22:errorcluster)
  n137 = VISA Close(VISA resource name=w5, error in (no error)=w4) -> ()  [unwired: 1 out]
  n138 = call "Destroy User Event - Stop.vi"("error in (no error)"=w22, "User Event - Stop"=w16) -> ("error out"=w19:errorcluster)  [unwired: 9 in]
  n139 = disable-structure shown="RUN_TIME_ENGINE==True" {
    disable-tunnel: w19 -> [_ _]
    frame condition #0 (active) {
    }
    frame condition #1 {
      # "Call Quit LabVIEW if running as a built application."
      n140 = Quit LabVIEW() -> ()  [unwired: 1 in]
    }
  }
